vi "SubVI Translate.vi"(8 "error in (no error)":errorcluster, 11 "SubVI in":refnum<vi>) -> (0 "error out":errorcluster, 2 "transcripted code":string, 3 "transcriptor cluster":T1)   [LabVIEW 2014]
uses:
  types/LabVIEW Universal Transcriptor Cluster.ctl
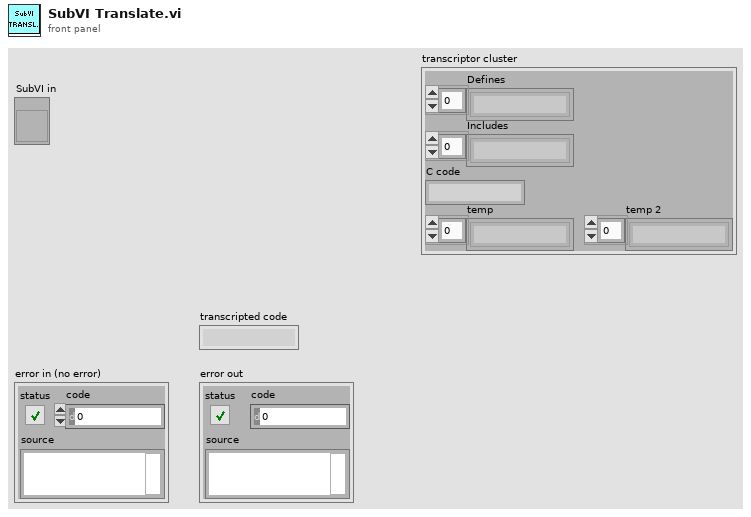
[diagram p1: front panel]
types:
  T1 = typedef "LabVIEW Universal Transcriptor Cluster.ctl" = cluster{"Defines":string[], "Includes":string[], "C code":string, "temp":string[], "temp 2":string[]}
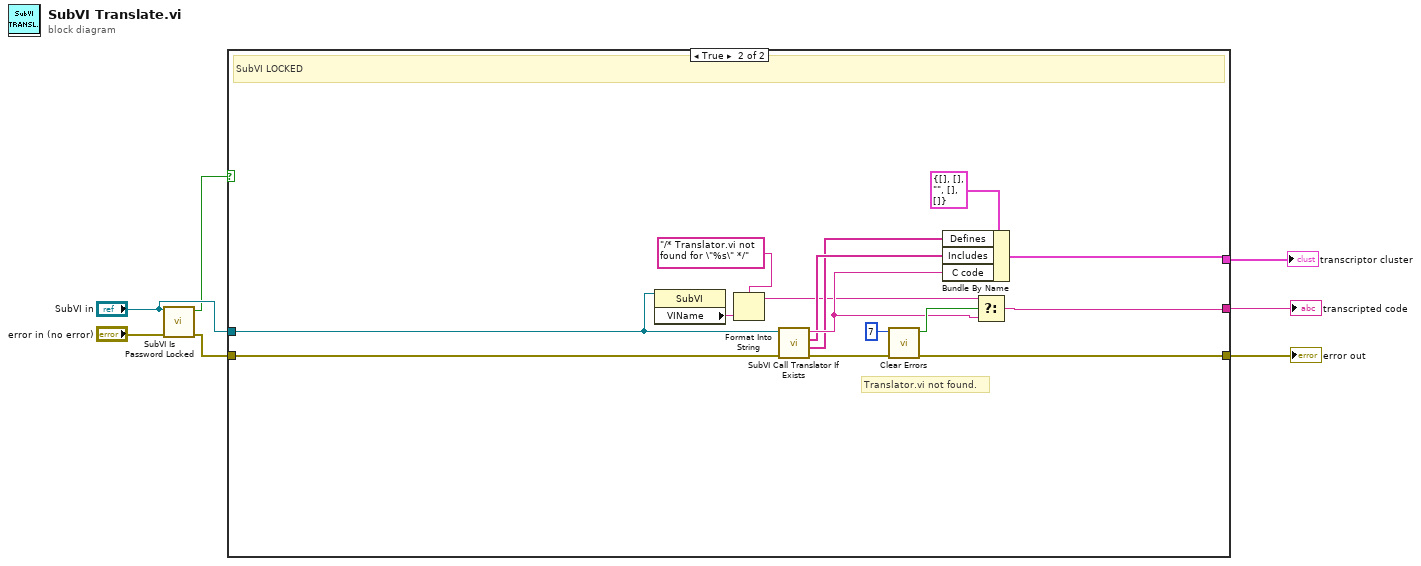
[diagram p0: block diagram]
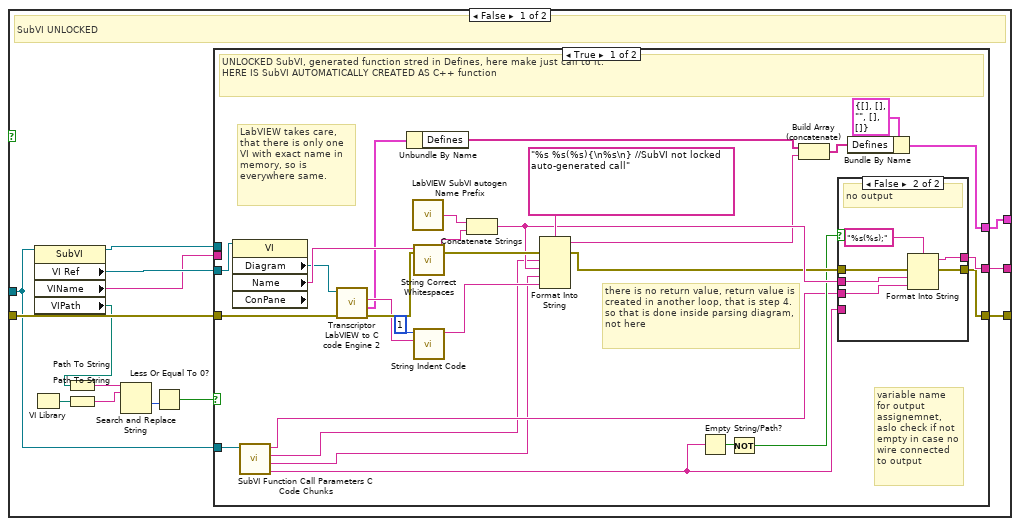
[diagram p2: hidden frame]
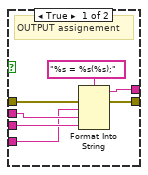
[diagram p3: hidden frame]
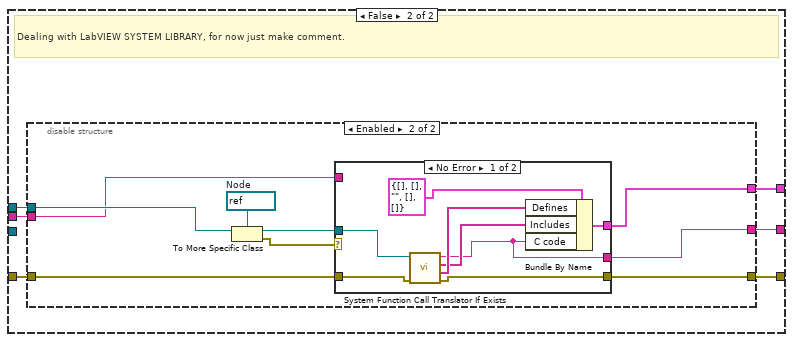
[diagram p4: hidden frame]
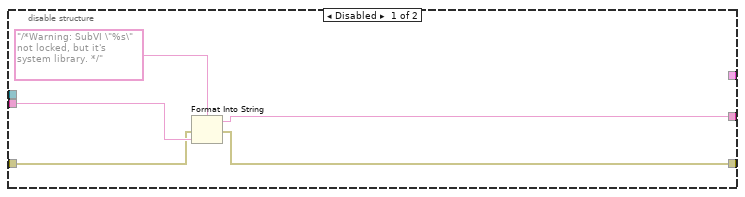
[diagram p5: hidden frame]
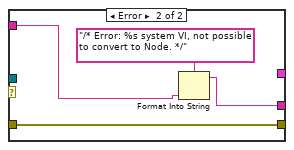
[diagram p6: hidden frame]
diagram:
  n1 = call "SubVI Is Password Locked.vi"("Error In"="error in (no error)", "SubVI ref"="SubVI in") -> ("Error Out"=w6:errorcluster, "isPasswordLocked?"=w2:bool)  [unwired: 8 in]
  n2 = case shown="True" w2 {
    tunnel: "SubVI in" -> [w9 w105]
    tunnel: [w19 w109] -> w4
    tunnel: w6 -> [w21 w108]
    tunnel: [w18 w107] -> w7
    tunnel: [w10 w106] -> w1
    frame False {
      # "SubVI UNLOCKED"
      n3 = VI Library() -> (path=w15:path)
      n4 = property class="SubVI"(reference=w9) -> (reference out=w8:refnum<vi>, "VI Ref"=w20:refnum<vi>, "VIName"=w17:string, "VIPath"=w16:path)  [unwired: 1 in, 1 out]
      n5 = Path To String(path=w16) -> (string=w14:string)
      n6 = Path To String(path=w15) -> (string=w13:string)
      n7 = Search and Replace String(input string=w14, search string=w13) -> (number of replacements=w12:i32)  [unwired: 6 in, 3 out]
      n8 = Less Or Equal To 0?(x=w12) -> (x <= 0?=w11:bool)
      n9 = case shown="True" w11 {
        tunnel: w21 -> [w49 w66]
        tunnel: w20 -> [w33 _]
        tunnel: [w47 w68] -> w19
        tunnel: [w35 w65] -> w18
        tunnel: w17 -> [_ w67]
        tunnel: [w48 w63] -> w10
        tunnel: w9 -> [w31 _]
        tunnel: w8 -> [_ w64]
        frame True {
          # "variable name for output assignemnet, aslo check if not empty in case no wire connected to output"
          # "there is no return value, return value is created in another loop, that is step 4.\nso that is done inside parsing diagram, not here"
          # "LabVIEW takes care, that there is only one VI with exact name in memory, so is everywhere same."
          # "UNLOCKED SubVI, generated function stred in Defines, here make just call to it.\nHERE IS SubVI AUTOMATICALLY CREATED AS C++ function"
          n10 = property class="VI" props=["Diagram", "Name", "ConPane"](reference=w33) -> ("Diagram"=w34:refnum<vi>, "Name"=w44:string)  [unwired: 1 in, 3 out]
          n11 = call "SubVI Function Call Parameters C Code Chunks.vi"("SubVI Refnum"=w31) -> ("SubVI output variable name"=w29:string, "SubVI func. declaration"=w22:string, "return datatype"=w23:string, "SubVI func. call in code"=w24:string)  [unwired: 5 in, 2 out]
          n12 = call "Transcriptor LabVIEW to C code Engine 2.vi"("Error In"=w49, "Diagram in"=w34) -> ("Error Out"=w45:errorcluster, "output cluster"=w27:T1, "transcripted code"=w43:string)  [unwired: 5 in, 2 out]
          n13 = Unbundle By Name(w27) -> ("Defines"=w26:string[])
          n14 = call "LabVIEW SubVI autogen Name Prefix.vi"() -> ("datatype prefix"=w41:string)
          n15 = call "String Correct Whitespaces.vi"("String in"=w44) -> ("String out"=w40:string)  [unwired: 10 in]
          n16 = call "String Indent Code.vi"("complete code"=w43, "actual nested level"=1) -> ("indented code"=w32:string)  [unwired: 9 in]
          n17 = Concatenate Strings(w41, w40) -> (w39:string)
          n18 = Format Into String(format string="%s %s(%s){\n%s\n} //SubVI not locked auto-generated call", error in=w45, w23, w39, w22, w32) -> (resulting string=w37:string, error out=w36:errorcluster)  [unwired: 1 in]
          n19 = Empty String/Path?(string/path=w29) -> (empty?=w30:bool)
          n20 = Not(x=w30) -> (.not. x?=w28:bool)
          n21 = Build Array (concatenate)(w26, w37) -> (w38:string[])
          n22 = case shown="False" w28 {
            tunnel: [w56 w62] -> w47
            tunnel: w39 -> [w54 w60]
            tunnel: w36 -> [w53 w59]
            tunnel: [w52 w58] -> w35
            tunnel: w24 -> [w51 w57]
            tunnel: w29 -> [w50 _]
            frame True {
              # "OUTPUT assignement"
              n23 = Format Into String(format string="%s = %s(%s);", error in=w53, w50, w54, w51) -> (resulting string=w56:string, error out=w52:errorcluster)  [unwired: 1 in]
            }
            frame False {
              # "no output"
              n24 = Format Into String(format string="%s(%s);", error in=w59, w60, w57) -> (resulting string=w62:string, error out=w58:errorcluster)  [unwired: 1 in]
            }
          }
          n25 = Bundle By Name(cluster=T1 {"Defines"=[], "Includes"=[], "C code"="", "temp"=[], "temp 2"=[]} ("input cluster"), "Defines"=w38) -> (w48:T1)
        }
        frame False {
          # "Dealing with LabVIEW SYSTEM LIBRARY, for now just make comment."
          n26 = disable-structure shown="Enabled" {
            disable-tunnel: [w72 w77] -> w68
            disable-tunnel: w67 -> [w71 w74]
            disable-tunnel: w66 -> [w70 w76]
            disable-tunnel: [w69 w82] -> w65
            disable-tunnel: w64 -> [_ w81]
            disable-tunnel: [_ w78] -> w63
            frame Disabled {
              n27 = Format Into String(format string="/*Warning: SubVI \"%s\" not locked, but it's system library. */", error in=w70, w71) -> (resulting string=w72:string, error out=w69:errorcluster)  [unwired: 1 in]
            }
            frame Enabled {
              w80 = refnum<vi> refnum  # Node
              n28 = To More Specific Class(target class=w80, reference=w81) -> (specific class reference=w79:refnum<vi>, error out=w75:errorcluster)  [unwired: 1 in]
              n29 = case shown="No Error" w75 {
                tunnel: [w90 w94] -> w82
                tunnel: w79 -> [w89 _]
                tunnel: [w86 _] -> w78
                tunnel: [w85 w91] -> w77
                tunnel: w76 -> [w84 w94]
                tunnel: w74 -> [_ w92]
                frame No Error {
                  n30 = call "System Function Call Translator If Exists.vi"("Error In"=w84, "Node Refnum"=w89) -> ("Error Out"=w90:errorcluster, "Defines"=w88:string[], "Includes"=w87:string[], "Replaced Code"=w85:string)  [unwired: 6 in]
                  n31 = Bundle By Name(cluster=T1 {"Defines"=[], "Includes"=[], "C code"="", "temp"=[], "temp 2"=[]} ("input cluster"), "Defines"=w88, "Includes"=w87, "C code"=w85) -> (w86:T1)
                }
                frame Error {
                  n32 = Format Into String(format string="/* Error: %s system VI, not possible to convert to Node. */" ("Replaced Code"), w92) -> (resulting string=w91:string)  [unwired: 2 in, 1 out]
                }
              }
            }
          }
        }
      }
    }
    frame True {
      # "Translator.vi not found."
      # "SubVI LOCKED"
      n33 = property class="SubVI"(reference=w105) -> ("VIName"=w98:string)  [unwired: 1 in, 2 out]
      n34 = Format Into String(format string="/* Translator.vi not found for \"%s\" */" ("t"), w98) -> (resulting string=w96:string)  [unwired: 2 in, 1 out]
      n35 = call "SubVI Call Translator If Exists.vi"("Error In"=w108, "SubVI Refnum"=w105) -> ("Error Out"=w104:errorcluster, "Defines"=w99:string[], "Includes"=w100:string[], "Replaced Code"=w101:string)  [unwired: 6 in]
      n36 = call <vilib>:"Clear Errors.vi"("error in (no error)"=w104, "specific error code to clear (0: all)"=7) -> ("error out"=w107:errorcluster, "specific error cleared?"=w102:bool)  [unwired: 4 in]
      n37 = Bundle By Name(cluster=T1 {"Defines"=[], "Includes"=[], "C code"="", "temp"=[], "temp 2"=[]} ("input cluster"), "Defines"=w99, "Includes"=w100, "C code"=w101) -> (w106:T1)
      n38 = Select(t=w96, s=w102, f=w101) -> (s? t:f=w109:string)
    }
  }
  "error out" <- w7
  "transcripted code" <- w4
  "transcriptor cluster" <- w1
